vi "Overlay Line with Arrows Simple.vi"(6 "Color":u32(colorbox)=16711680, 7 "Group":string, 8 "error in":errorcluster, 9 "Arrows":cluster{"Start point":bool, "End point":bool}, 10 "Line Coordinates":T1, 11 "Image In":T2) -> (0 "error out":errorcluster, 3 "Image Out":T2)   [LabVIEW 2016]
uses:
  <vilib>/vision/Image Controls.llb/IMAQ Image.ctl
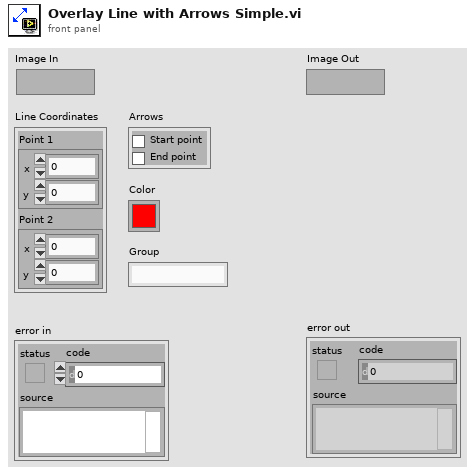
[diagram p1: front panel]
types:
  T1 = cluster{"Point 1":cluster{"x":dbl, "y":dbl}, "Point 2":cluster{"x":dbl, "y":dbl}}
  T2 = typedef "IMAQ Image.ctl" = refnum<image>
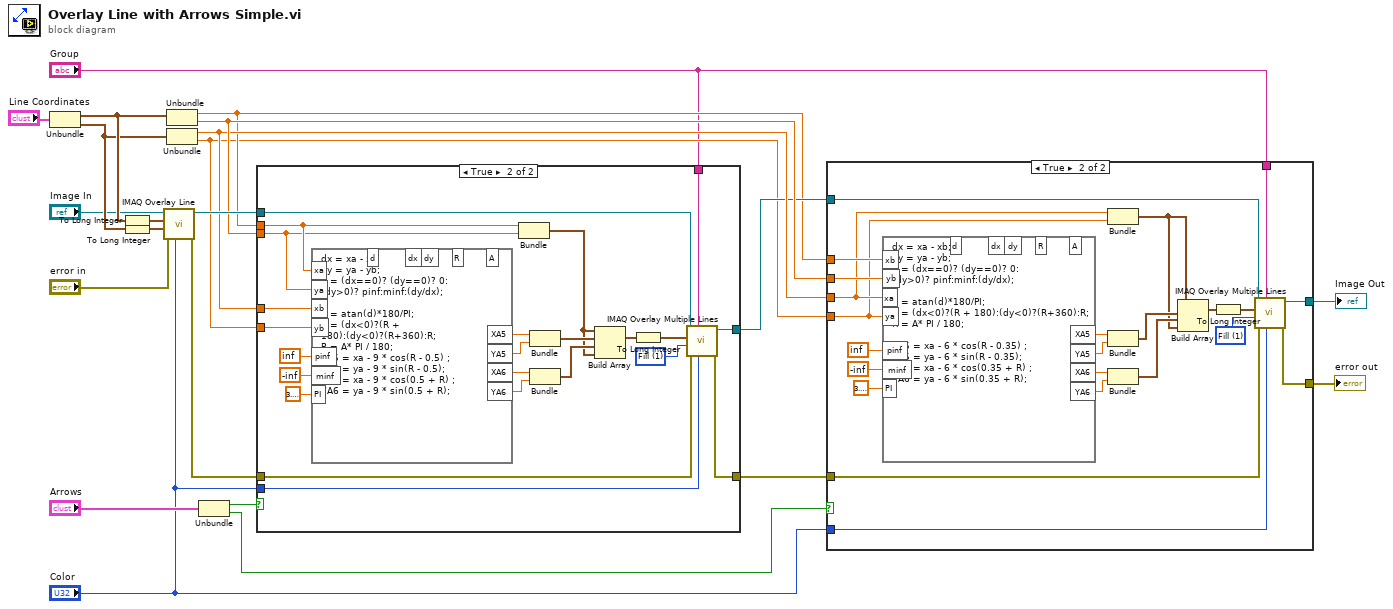
[diagram p0: block diagram]
diagram:
  n1 = Unbundle("Line Coordinates") -> ("Point 1"=w14:cluster{"x":dbl, "y":dbl}, "Point 2"=w13:cluster{"x":dbl, "y":dbl})
  n2 = To Long Integer(number=w14) -> (32bit integer=w12:cluster{"x":i32, "y":i32})
  n3 = To Long Integer(number=w13) -> (32bit integer=w11:cluster{"x":i32, "y":i32})
  n4 = call "IMAQ Overlay Line"("Color"="Color", "error in (no error)"="error in", "End Point"=w11, "Start Point"=w12, "Image"="Image In") -> ("error out"=w7:errorcluster, "Image Out"=w22:T2)  [unwired: 1 in, 4 out]
  n5 = Unbundle(w14) -> ("x"=w10:dbl, "y"=w20:dbl)
  n6 = Unbundle(w13) -> ("x"=w19:dbl, "y"=w9:dbl)
  n7 = Unbundle("Arrows") -> ("Start point"=w17:bool, "End point"=w1:bool)
  n8 = case shown="True" w17 {
    tunnel: w10 -> [_ w36]
    tunnel: w20 -> [_ w35]
    tunnel: w19 -> [_ w37]
    tunnel: w9 -> [_ w34]
    tunnel: w22 -> [w24 w33]
    tunnel: [w24 w31] -> w15
    tunnel: "Color" -> [_ w30]
    tunnel: w7 -> [w23 w27]
    tunnel: [w23 w26] -> w6
    tunnel: "Group" -> [_ w25]
    frame False {
    }
    frame True {
      w29 = u32 1 items=["Frame", "Fill"] ("Drawing Mode (Frame)")
      n9 = formula code="dx = xa - xb;\ndy = ya - yb;\nd = (dx==0)? (dy==0)? 0: \n(dy>0)? pinf:minf:(dy/dx);\n\nR = atan(d)*180/PI;\nA = (dx<0)?(R + 180):(dy<0)?(R+360):R;\nR = A* PI / 180;\nXA5 = xa - 9 * cos(R - 0.5) ;\nYA5 = ya - 9 * sin(R - 0.5);\nXA6 = xa - 9 * cos(0.5 + R) ;\nYA6 = ya - 9 * sin(0.5 + R);"("xa"=w36, "ya"=w35, "xb"=w37, "yb"=w34, "pinf"=inf, "minf"=-inf, "PI"=3.141592653589793) -> ("XA5"=w44:dbl, "YA5"=w43:dbl, "XA6"=w42:dbl, "YA6"=w41:dbl)  [unwired: 5 out]
      n10 = Bundle("x"=w36, "y"=w35) -> (w38:cluster{"x":dbl, "y":dbl})  [unwired: 1 out]
      n11 = Bundle("XA5"=w44, "YA5"=w43) -> (w40:cluster{"XA5":dbl, "YA5":dbl})  [unwired: 1 out]
      n12 = Bundle("XA6"=w42, "YA6"=w41) -> (w39:cluster{"XA6":dbl, "YA6":dbl})  [unwired: 1 out]
      n13 = Build Array(w38, w40, w39, w38) -> (w32:cluster{"x":dbl, "y":dbl}[])
      n14 = To Long Integer(number=w32) -> (32bit integer=w28:cluster{"x":i32, "y":i32}[])
      n15 = call "IMAQ Overlay Multiple Lines"("Color"=w30, "Group"=w25, "error in (no error)"=w27, "Drawing Mode (Frame)"=w29, "Line End Points"=w28, "Image"=w33) -> ("error out"=w26:errorcluster, "Image Out"=w31:T2)  [unwired: 4 out]
    }
  }
  n16 = case shown="True" w1 {
    tunnel: w10 -> [_ w69]
    tunnel: w20 -> [_ w68]
    tunnel: w19 -> [_ w67]
    tunnel: w9 -> [_ w66]
    tunnel: w15 -> [w49 w57]
    tunnel: [w49 w56] -> w16
    tunnel: "Color" -> [_ w55]
    tunnel: w6 -> [w48 w52]
    tunnel: [w48 w51] -> w5
    tunnel: "Group" -> [_ w50]
    frame False {
    }
    frame True {
      w54 = u32 1 items=["Frame", "Fill"] ("Drawing Mode (Frame)")
      n17 = formula code="dx = xa - xb;\ndy = ya - yb;\nd = (dx==0)? (dy==0)? 0:\n(dy>0)? pinf:minf:(dy/dx);\n\nR = atan(d)*180/PI;\nA = (dx<0)?(R + 180):(dy<0)?(R+360):R;\nR = A* PI / 180;\n\nXA5 = xa - 6 * cos(R - 0.35) ;\nYA5 = ya - 6 * sin(R - 0.35);\nXA6 = xa - 6 * cos(0.35 + R) ;\nYA6 = ya - 6 * sin(0.35 + R);"("xb"=w69, "yb"=w68, "xa"=w67, "ya"=w66, "pinf"=inf, "minf"=-inf, "PI"=3.141592653589793) -> ("XA5"=w65:dbl, "YA5"=w64:dbl, "XA6"=w63:dbl, "YA6"=w62:dbl)  [unwired: 5 out]
      n18 = Bundle("x"=w67, "y"=w66) -> (w59:cluster{"x":dbl, "y":dbl})  [unwired: 1 out]
      n19 = Bundle("XA5"=w65, "YA5"=w64) -> (w61:cluster{"XA5":dbl, "YA5":dbl})  [unwired: 1 out]
      n20 = Bundle("XA6"=w63, "YA6"=w62) -> (w60:cluster{"XA6":dbl, "YA6":dbl})  [unwired: 1 out]
      n21 = Build Array(w59, w61, w60, w59) -> (w58:cluster{"x":dbl, "y":dbl}[])
      n22 = To Long Integer(number=w58) -> (32bit integer=w53:cluster{"x":i32, "y":i32}[])
      n23 = call "IMAQ Overlay Multiple Lines"("Color"=w55, "Group"=w50, "error in (no error)"=w52, "Drawing Mode (Frame)"=w54, "Line End Points"=w53, "Image"=w57) -> ("error out"=w51:errorcluster, "Image Out"=w56:T2)  [unwired: 4 out]
    }
  }
  "Image Out" <- w16
  "error out" <- w5
